vi "Initial State + LabVIEW Support.vi"() -> ()   [LabVIEW 2018]
doc: "This VI is placed in the LabVIEW Help menu to give a link to Initial State detailed Help"
uses:
  <vilib>/Platform/browser.llb/Open URL in Default Browser (string).vi
panel:
  in  "Debug":bool
  in  "Cancel":bool
  in  "Online Help Available  (Click Below)":bool
  # "Online Help and Email Support Available (Click Below)"
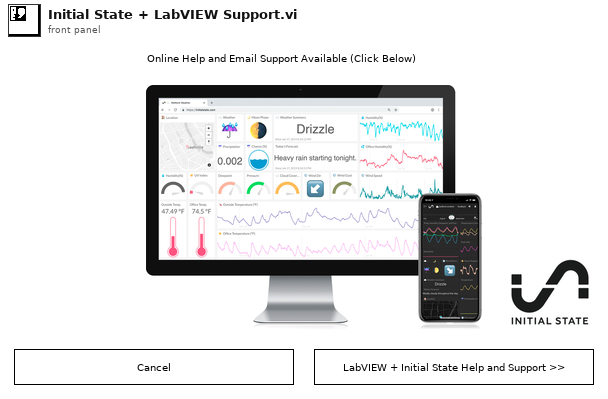
[diagram p1: front panel]
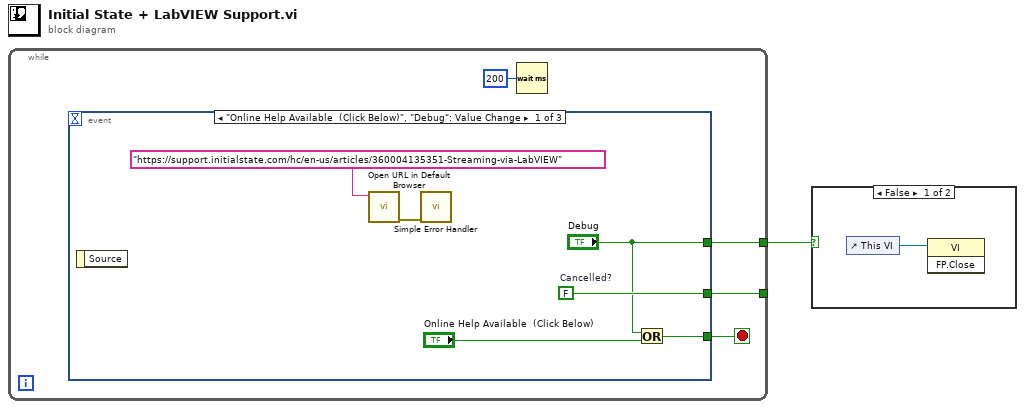
[diagram p0: block diagram]
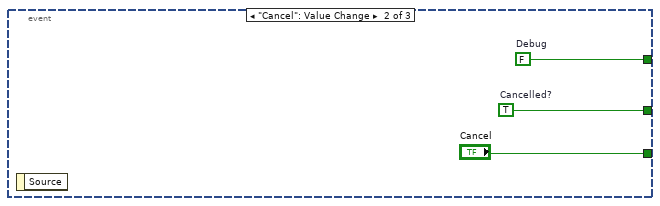
[diagram p3: hidden frame]
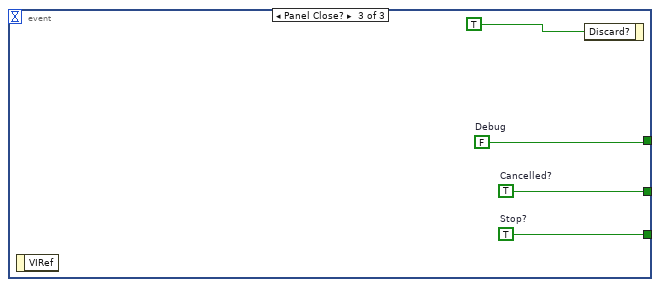
[diagram p4: hidden frame]
diagram:
  n1 = while {
    tunnel: [w4] -> _
    tunnel: [w2] -> w1
    stop <- w5 stop-if-true
    n2 = event shown="[0] \"Online Help Available  (Click Below)\", \"Debug\": Value Change" {
      selector: _ -> [_ _ _]
      dyn-events: _ -> [_ _ _]
      timeout: _ -> [_ _ _]
      tunnel: [w6 "Cancel" w17] -> w5
      tunnel: [w11 w14 w16] -> w4
      tunnel: ["Debug" w12 w15] -> w2
      event "Online Help Available  (Click Below)", "Debug": Value Change {
        w11 = FALSE  # Cancelled?
        n3 = event-data() -> ()  [unwired: 1 in, 1 out]
        n4 = call-poly <vilib>:"Open URL in Default Browser.vi"("URL"="https://support.initialstate.com/hc/en-us/articles/360004135351-Streaming-via-LabVIEW" ("Help URL")) -> ("error out"=w10:errorcluster)  [unwired: 5 in, 1 out]
        n5 = call <vilib>:"Simple Error Handler.vi"("error in (no error)"=w10) -> ()  [unwired: 4 in, 5 out]
        n6 = Or(x="Debug", y="Online Help Available  (Click Below)") -> (x .or. y?=w6:bool)
      }
      event "Cancel": Value Change {
        w12 = FALSE  # Debug
        w14 = TRUE  # Cancelled?
        n7 = event-data() -> ()  [unwired: 1 in, 1 out]
      }
      event Panel Close? {
        w15 = FALSE  # Debug
        w16 = TRUE  # Cancelled?
        w17 = TRUE  # Stop?
        n8 = event-data() -> ()  [unwired: 1 in, 1 out]
        n9 = event-data("Discard?"=TRUE) -> ()  [unwired: 1 in, 1 out]
      }
    }
    n10 = Wait (ms)(milliseconds to wait=u32 200) -> ()  [unwired: 1 out]
  }
  n11 = case shown="False" w1 {
    frame False {
      n12 = control-ref of="This VI"() -> (w19:refnum<vi>)
      n13 = invoke class="VI" method="FP.Close"(reference=w19) -> ()  [unwired: 2 in, 3 out]
    }
    frame True {
    }
  }
